vi "PolyCreate.vi"() -> ()   [LabVIEW 2020]
uses:
  <vilib>/Utility/miscctls.llb/LVMapReplaceAction.ctl
  269c9377-1933-43b6-923f-e4fc9fbce505.vi
  <vilib>/Comparison/Equal/Equal Functor/Equal Functor.lvclass
  <vilib>/regexp/Match Regular Expression.xnode
panel:
  out "error out":errorcluster
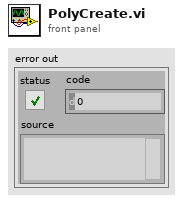
[diagram p1: front panel]
types:
  T1 = typedef "LVMapReplaceAction.ctl" = enum32{"Modify Entry only if found", "Add or Modify Entry", "Delete Entry"}
  T2 = enum32{"invalid VI type", "Standard VI", "Control VI", "Global VI", "Polymorphic VI", "Configuration VI", "SubSystem", "Facade VI", "Method VI", "Statechart Diagram VI"}
  T3 = cluster{"VIPath":path, "Menu Name":string, "Selector Name":string}
  T4 = cluster{"VIPath":path, "Menu Name":string, "Selector Name":string}[]
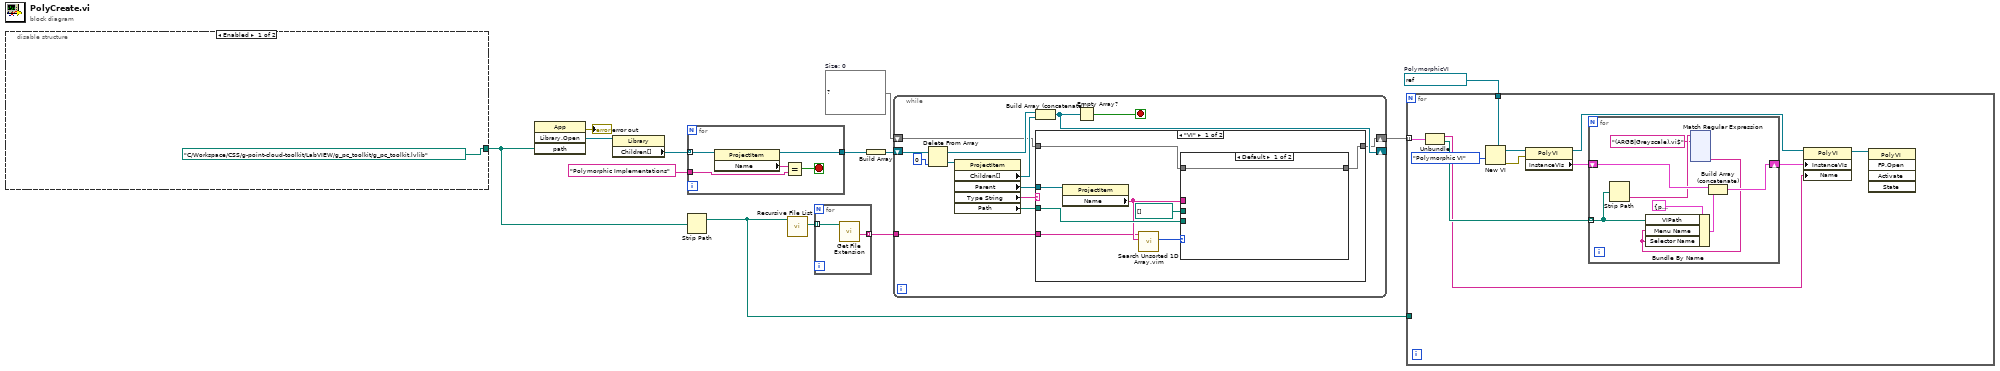
[diagram p0: block diagram]
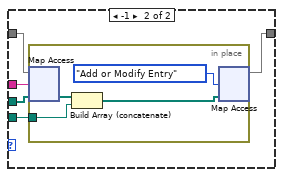
[diagram p3: hidden frame]
diagram:
  w2 = refnum<vi> refnum  # PolymorphicVI
  w8 = map{string, path[]} {}  # Size: 0
  n1 = disable-structure shown="Enabled" {
    disable-tunnel: [path "C:/Workspace/CSS/g-point-cloud-toolkit/LabVIEW/g_pc_toolkit/g_pc_toolkit.lvlib" ("Path") _] -> w7
    frame Enabled {
    }
    frame Disabled {
    }
  }
  n2 = invoke class="App" method="Library.Open"("path"=w7) -> (error out=→"error out":errorcluster, "Open Library"=w13:refnum<vi>)  [unwired: 3 in, 2 out]
  n3 = property class="Library"(reference=w13) -> ("Children[]"=w12:refnum<vi>[])  [unwired: 1 in, 2 out]
  n4 = for {
    tunnel: w12 -> [w19] mode=indexing
    tunnel: [w18] -> w11
    tunnel: "Polymorphic Implementations" ("y") -> [w16]
    stop <- w15 stop-if-true
    n5 = property class="ProjectItem"(reference=w19) -> (reference out=w18:refnum<vi>, "Name"=w17:string)  [unwired: 1 in, 1 out]
    n6 = Equal?(x=w17, y=w16) -> (x = y?=w15:bool)
  }
  n7 = Strip Path(path=w7) -> (stripped path=w3:path)  [unwired: 1 out]
  n8 = call <vilib>:"Recursive File List.vi"("Folder Path"=w3) -> ("All Files in Dir"=w6:path[])  [unwired: 6 in, 4 out]
  n9 = for {
    tunnel: w6 -> [w21] mode=indexing
    tunnel: [w20] -> w5 mode=indexing
    n10 = call <vilib>:"Get File Extension.vi"("file"=w21) -> ("filename without extension"=w20:string)  [unwired: 6 in, 4 out]
  }
  n11 = Build Array(w11) -> (w10:refnum<vi>[])
  n12 = while {
    shift-right: [w30] -> _
    shift-left: w10 -> [w34]
    shift-right: [w24] -> w4
    shift-left: w8 -> [w23]
    tunnel: w5 -> [w22]
    stop <- w29 stop-if-true
    n13 = Delete From Array(array=w34, index=0) -> (deleted portion=w32:refnum<vi>, array with subset deleted=w31:refnum<vi>[])  [unwired: 1 in]
    n14 = property class="ProjectItem"(reference=w32) -> ("Children[]"=w27:refnum<vi>[], "Parent"=w26:refnum<vi>, "Type String"=w28:string, "Path"=w25:path)  [unwired: 1 in, 2 out]
    n15 = Build Array (concatenate)(w31, w27) -> (w30:refnum<vi>[])
    n16 = case shown="\"VI\"" w28 {
      tunnel: w26 -> [w42 _]
      tunnel: w25 -> [w40 _]
      tunnel: [w39 w53] -> w24
      tunnel: w23 -> [w38 w53]
      tunnel: w22 -> [w36 _]
      frame "VI" {
        n17 = property class="ProjectItem"(reference=w42) -> ("Name"=w37:string)  [unwired: 1 in, 2 out]
        n18 = call "Search Unsorted 1D Array.vim"("element"=w37, "unsorted 1D array"=w36) -> ("index of element"=w35:i32)  [unwired: 9 in]
        n19 = case shown="Default" w35 {
          tunnel: path[] [] -> [_ w48]
          tunnel: w40 -> [_ w47]
          tunnel: [w43 w46] -> w39
          tunnel: w38 -> [w43 w45]
          tunnel: w37 -> [_ w44]
          frame Default {
          }
          frame -1 {
            n20 = in-place {
              in-place-border: w47 -> [w51]
              n21 = in-place-map #1(w45, w44, w48) -> (w52:path[])  [unwired: 1 out]
              n22 = Build Array (concatenate)(w52, w51) -> (w50:path[])
              n23 = in-place-map #1(w50, LVMapReplaceAction."Add or Modify Entry" ("action")) -> (w46:map{string, path[]})  [unwired: 2 out]
            }
          }
        }
      }
      frame Default {
      }
    }
    n24 = Empty Array?(array=w30) -> (empty?=w29:bool)
  }
  n25 = for {
    tunnel: w4 -> [w64] mode=indexing
    tunnel: w2 -> [w63]
    tunnel: w3 -> [_]
    n26 = Unbundle(w64) -> ("Name"=w56:string, w59:path[])
    n27 = New VI(5:w63, 9:T2."Polymorphic VI" ("vi type (standard vi)")) -> (0:w61:errorcluster, 3:w62:refnum<vi>)  [unwired: 5 in]
    n28 = property class="PolyVI"(reference=w62, error in=w61) -> (reference out=w57:refnum<vi>, "InstanceVIs"=w60:T4)  [unwired: 1 out]
    n29 = for {
      shift-right: [w71] -> w58
      shift-left: w60 -> [w72]
      tunnel: w59 -> [w68] mode=indexing
      n30 = Strip Path(path=w68) -> (name=w67:string)  [unwired: 1 out]
      n31 = xnode "Match Regular Expression"("input string"=w67, "regular expression"="(ARGB|Greyscale).vi$") -> ("submatch 1"=w65:string)  [unwired: 4 in, 5 out]
      n32 = Bundle By Name(cluster=T3 {"VIPath"=path "", "Menu Name"="", "Selector Name"=""}, "VIPath"=w68, "Menu Name"=w65, "Selector Name"=w65) -> (w69:T3)
      n33 = Build Array (concatenate)(w72, w69) -> (w71:T4)
    }
    n34 = property class="PolyVI"(reference=w57, "InstanceVIs"=w58, "Name"=w56) -> (reference out=w55:refnum<vi>)  [unwired: 1 in, 1 out]
    n35 = invoke class="PolyVI" method="FP.Open"(reference=w55) -> ()  [unwired: 4 in, 5 out]
  }
